vi "Init_Open_Close.vi"(6 "pattern":string, 8 "error in":errorcluster, 10 "path to start the search":path, 11 "Tree In":refnum<vi>) -> (0 "error out":errorcluster, 1 "Number of files found":i32, 3 "Tree Out":refnum<vi>)   [LabVIEW 2012]
doc: "This VI first clears the tree control. After the tree control is populated, it closes all the \"children\" in the tree control."
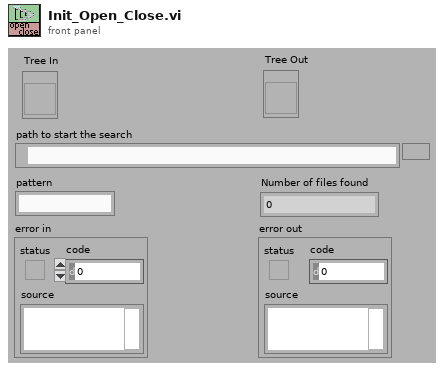
[diagram p1: front panel]
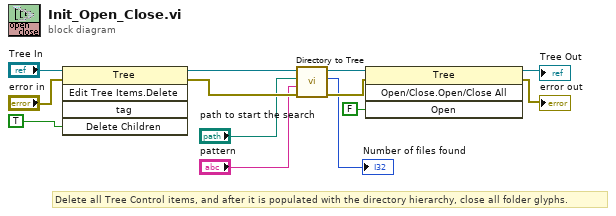
[diagram p0: block diagram]
diagram:
  # "Delete all Tree Control items, and after it is populated with the directory hierarchy, close all folder glyphs."
  n1 = invoke on="Invoke Node" class="Tree" method="Edit Tree Items.Delete"(reference="Tree In", error in="error in", "Delete Children"=TRUE ("Open")) -> (reference out=w10:refnum<vi>, error out=w9:errorcluster)  [unwired: 2 in, 3 out]
  n2 = call "Directory to Tree.vi"("error in"=w9, "Pattern"="pattern", "Path to start the search"="path to start the search", "Tree In"=w10) -> ("error out"=w5:errorcluster, "Number of files found"=→"Number of files found":i32, "Tree Out"=w6:refnum<vi>)  [unwired: 2 in, 1 out]
  n3 = invoke on="Invoke Node" class="Tree" method="Open/Close.Open/Close All"(reference=w6, error in=w5, "Open"=FALSE) -> (reference out=→"Tree Out":refnum<vi>, error out=→"error out":errorcluster)  [unwired: 1 in, 2 out]
